vi "Extract Sclera Plane.vi"(8 "error in (no error)":errorcluster, 10 "target":T1, 11 "source":T1) -> (0 "error out":errorcluster, 2 "Array":u8[][](array[numeric]), 3 "target":T1)   [LabVIEW 2014]
doc: "Extracts the sclera plane and puts it into the specified buffer image."
uses:
  <vilib>/vision/Image Controls.llb/IMAQ Image.ctl
  <vilib>/vision/NI_Vision_Development_Module.lvlib
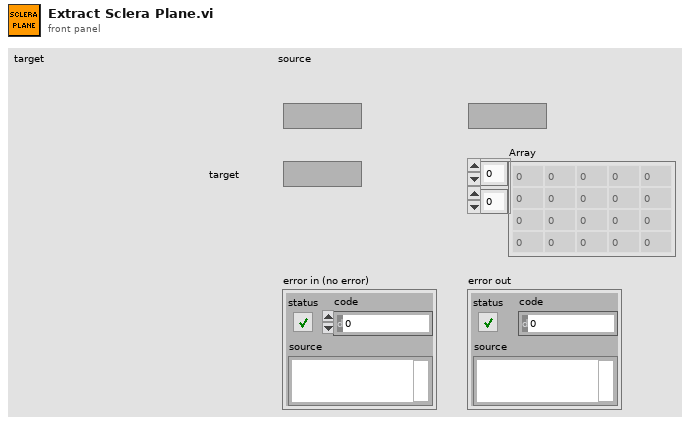
[diagram p1: front panel]
types:
  T1 = typedef "IMAQ Image.ctl" = refnum<image>
  T2 = cluster{"Red (or Hue) value":u8, "Green (or Sat) value":u8, "Blue (or Light or Val) value":u8}[][]
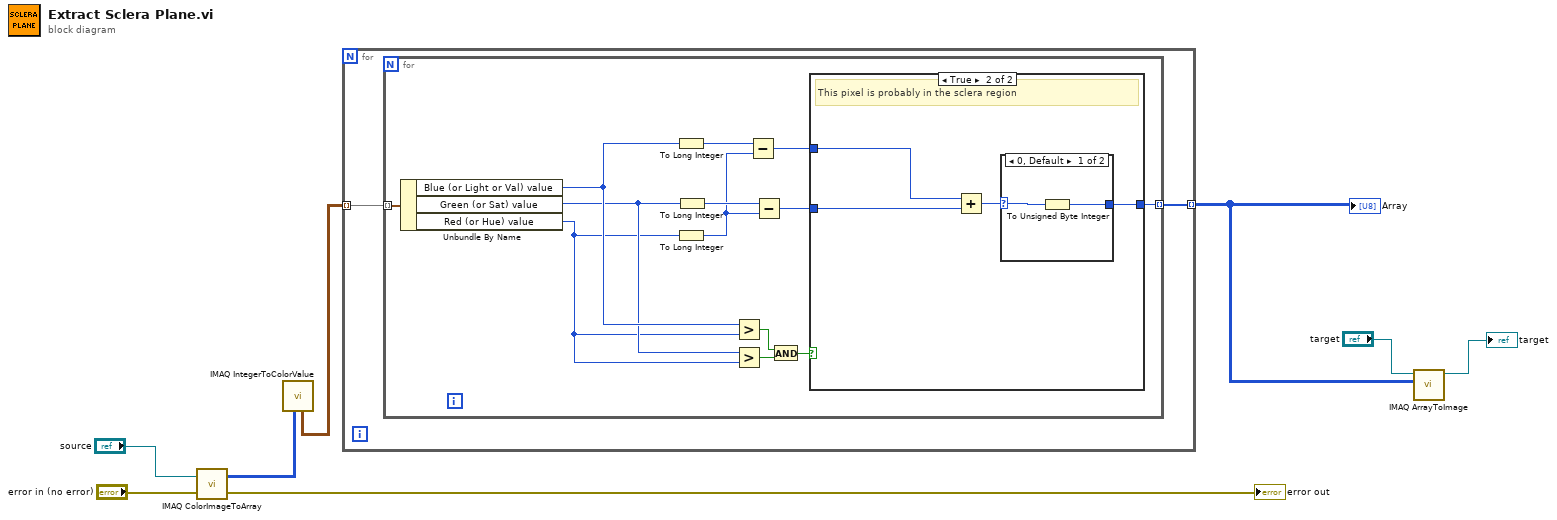
[diagram p0: block diagram]
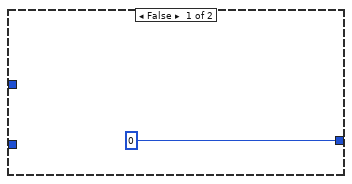
[diagram p2: hidden frame]
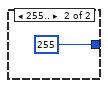
[diagram p3: hidden frame]
diagram:
  n1 = call "IMAQ ColorImageToArray"("Image"="source", "error in (no error)"="error in (no error)") -> ("Image Pixels (U32)"=w5:u32[][], "error out"=→"error out":errorcluster)  [unwired: 2 in, 1 out]
  n2 = call "IMAQ IntegerToColorValue"("2D U32 array"=w5) -> ("2D Color value array"=w6:T2)  [unwired: 4 in, 3 out]
  n3 = for {
    tunnel: w6 -> [w10] mode=indexing
    tunnel: [w9] -> w7 mode=indexing
    n4 = for {
      tunnel: w10 -> [w23] mode=indexing
      tunnel: [w22] -> w9 mode=indexing
      n5 = Unbundle By Name(w23) -> ("Blue (or Light or Val) value"=w13:u8, "Green (or Sat) value"=w12:u8, "Red (or Hue) value"=w11:u8)
      n6 = To Long Integer(number=w13) -> (32bit integer=w18:i32)
      n7 = To Long Integer(number=w11) -> (32bit integer=w16:i32)
      n8 = To Long Integer(number=w12) -> (32bit integer=w17:i32)
      n9 = Greater?(x=w13, y=w11) -> (0:w20:bool)
      n10 = Greater?(x=w12, y=w11) -> (0:w19:bool)
      n11 = Subtract(x=w18, y=w16) -> (x-y=w15:i32)
      n12 = Subtract(x=w17, y=w16) -> (x-y=w14:i32)
      n13 = And(x=w20, y=w19) -> (x .and. y?=w21:bool)
      n14 = case shown="True" w21 {
        tunnel: [u8 0 w25] -> w22
        tunnel: w15 -> [_ w27]
        tunnel: w14 -> [_ w28]
        frame False {
        }
        frame True {
          # "This pixel is probably in the sclera region"
          n15 = Add(x=w27, y=w28) -> (x+y=w26:i32)
          n16 = case shown="0, Default" w26 {
            selector: w26 -> [w30 _]
            tunnel: [w29 u8 255] -> w25
            frame 0, Default {
              n17 = To Unsigned Byte Integer(number=w30) -> (unsigned 8bit integer=w29:u8)
            }
            frame 255.. {
            }
          }
        }
      }
    }
  }
  "Array" <- w7
  n18 = call "IMAQ ArrayToImage"("Image Pixels (U8)"=w7, "Image"="target") -> ("Image Out"=→"target":T1)  [unwired: 8 in, 1 out]
